vi "Set Tree Data Definitions.vi"(8 "Error In":errorcluster, 10 "Tree Data Defs":refnum<class "Tree Data.lvclass">[](array[class]), 11 "Tree Manager":T1) -> (0 "Error Out":errorcluster, 3 "Tree Manager":T1)   [LabVIEW 2020, in "NI_VIAnCFGDataStructure.lvlib" / "Tree.lvclass"]
doc: "Set the definitions of Tree Data classes used to recognize, flatten and unflatten XML and LV Tree Control data.\n\n<b>WARNING</b> Only use this method if you are sure what you are doing. This overwrites default classes used to understand Tree Data types."
uses:
  <vilib>/addons/analyzer/VIAnCFGDataStructure/Tree Manager/Tree.lvclass
  <vilib>/addons/analyzer/VIAnCFGDataStructure/Tree Manager/Typedefs/Session Handle.ctl
  <vilib>/addons/analyzer/VIAnCFGDataStructure/Tree Data/Tree Data.lvclass
  <vilib>/addons/analyzer/VIAnCFGDataStructure/Tree Manager/Tree.lvclass/Tree.ctl
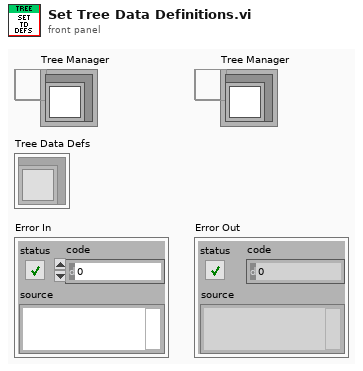
[diagram p1: front panel]
types:
  T1 = typedef "NI_VIAnCFGDataStructure.lvlib/Tree.lvclass/Session Handle.ctl" = refnum<data-value>
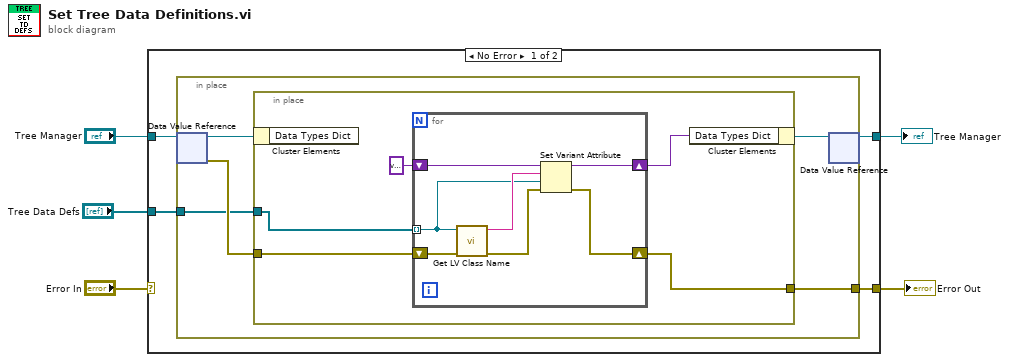
[diagram p0: block diagram]
diagram:
  n1 = case shown="No Error" "Error In" {
    selector: "Error In" -> [_ w27]
    tunnel: "Tree Manager" -> [w9 w28]
    tunnel: [w8 w28] -> w4
    tunnel: [w7 w27] -> w2
    tunnel: "Tree Data Defs" -> [w6 _]
    frame No Error {
      n2 = in-place {
        in-place-border: [w13] -> w7
        in-place-border: w6 -> [w10]
        n3 = in-place-dvr #1(w9) -> (w14:refnum<class "Tree.lvclass">, w11:errorcluster)
        n4 = in-place {
          in-place-border: [w16] -> w13
          in-place-border: w11 -> [w19]
          in-place-border: w10 -> [w18]
          n5 = in-place-cluster #2(w14) -> ()  [unwired: 1 out]
          n6 = for {
            shift-right: [w25] -> w17
            shift-left: variant ("Tree Dictionary") -> [w26]
            tunnel: w18 -> [w23] mode=indexing
            shift-right: [w20] -> w16
            shift-left: w19 -> [w22]
            n7 = call <vilib>:"Get LV Class Name.vi"("error in (no error)"=w22, "object"=w23) -> ("error out"=w21:errorcluster, "class name"=w24:string)  [unwired: 8 in]
            n8 = Set Variant Attribute(Variant=w26, name=w24, value=w23, error in=w21) -> (Variant out=w25:variant, error out=w20:errorcluster)  [unwired: 1 out]
          }
          n9 = in-place-cluster #2("Data Types Dict"=w17) -> (w12:refnum<class "Tree.lvclass">)
        }
        n10 = in-place-dvr #1(w12) -> (w8:T1)  [unwired: 1 out]
      }
    }
    frame Error {
    }
  }
  "Tree Manager" <- w4
  "Error Out" <- w2
